vi "Assemble-image-arrays.vi"(8 "error in":errorcluster, 11 "Image sizes":u32[][](array[numeric])) -> (0 "error IO":errorcluster, 3 "Zero images":i8[][][](array[numeric]))   [LabVIEW 2013, in "CameraVision.lvlib" / "CV-Configuration.lvclass"]
uses:
  CV-Configuration.lvclass
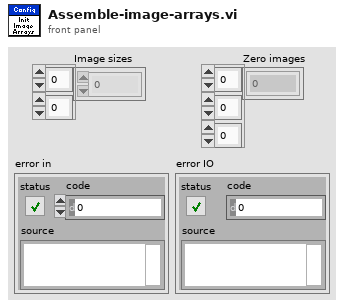
[diagram p1: front panel]
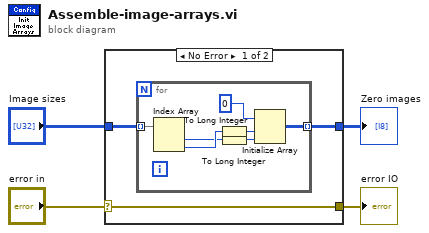
[diagram p0: block diagram]
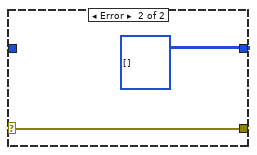
[diagram p2: hidden frame]
diagram:
  n1 = case shown="No Error" "error in" {
    selector: "error in" -> [w6 w16]
    tunnel: "Image sizes" -> [w7 _]
    tunnel: [w6 w16] -> w2
    tunnel: [w5 i8[][][] []] -> w1
    frame No Error {
      n2 = for {
        tunnel: w7 -> [w13] mode=indexing
        tunnel: [w12] -> w5 mode=indexing
        n3 = Index Array(array=w13) -> (element #1=w10:u32, element #2=w11:u32)  [unwired: 2 in]
        n4 = To Long Integer(number=w11) -> (32bit integer=w9:i32)
        n5 = To Long Integer(number=w10) -> (32bit integer=w8:i32)
        n6 = Initialize Array(i8 0, w9, w8) -> (w12:i8[][])
      }
    }
    frame Error {
    }
  }
  "Zero images" <- w1
  "error IO" <- w2
